vi "Get DDG Lite Pulses Per Exposure.vi"(10 "ui32Pulses":u32, 11 "channel":u32(ring)=65535 items=["AT_DDGLite_ChannelA"=1073741824, "AT_DDGLite_ChannelB"=1073741825, "AT_DDGLite_ChannelC"=1073741826]) -> (2 "ui32Pulses out":u32, 3 "function return":u32)   [LabVIEW 2018, in "Copy of Andor SDK.lvlib"]
doc: "EXPNETTYPE unsigned int WINAPI GetDDGLitePulsesPerExposure(AT_DDGLiteChannelId channel, at_u32 * ui32Pulses);"
uses:
  Copy of Andor SDK.lvlib
  <userlib>/Andor SDK/ATMCD32D.dll
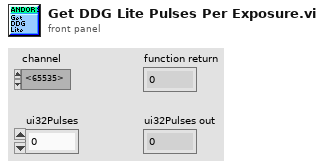
[diagram p1: front panel]
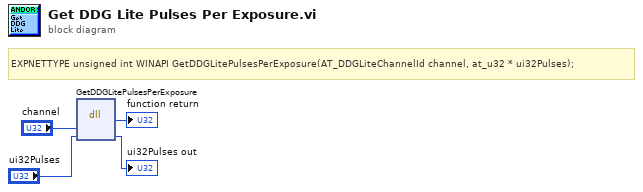
[diagram p0: block diagram]
diagram:
  # "EXPNETTYPE unsigned int WINAPI GetDDGLitePulsesPerExposure(AT_DDGLiteChannelId channel, at_u32 * ui32Pulses);"
  n1 = dll-call lib="C:/Program Files (x86)/National Instruments/LabVIEW 2018/user.lib/Andor SDK/ATMCD32D.*" fn="GetDDGLitePulsesPerExposure"("channel"="channel", "ui32Pulses"="ui32Pulses") -> (→"function return":u32, "ui32Pulses"=→"ui32Pulses out":u32)  [unwired: 4 in, 2 out]
